vi "Legend Palette.vi"(4 "Active Plot":i32, 6 "Control Ref Queue":T4, 9 "Window Bounds":T5, 10 "Multiplot Representation In":T1, 11 "2D Compass.lvclass in":refnum<class "2D Compass.lvclass">) -> (1 "Cancel?":bool, 2 "Multiplot Representation Out":T1, 3 "2D Compass.lvclass out":refnum<class "2D Compass.lvclass">)   [LabVIEW 2017, in "2D Compass.lvclass"]
uses:
  <vilib>/Math Plots/2D Math Plots/2D Compass/2D Compass/2D Compass.lvclass
  e:/builds/penguin/labview/branches/2017/dev/dist/vi.lib/Math Plots/2D Math Plots/2D Plot/2D Plot/2D Plot.lvclass
  <vilib>/Math Plots/2D Math Plots/2D Plot/Action String/2DMathPlot Ctrl Act Queue.ctl
  <vilib>/Math Plots/2D Math Plots/2D Plot/Action String/2DMathPlot Ctrl Act Cluster.ctl
  <vilib>/Math Plots/2D Math Plots/2D Plot/Action String/2DMathPlot State Class.ctl
  <vilib>/Math Plots/2D Math Plots/2D Plot/2D Plot/Typedef/Multiplot Representation.ctl
  <vilib>/Math Plots/2D Math Plots/2D Plot/2D Plot/Typedef/Plot Representation.ctl
  <vilib>/Math Plots/2D Math Plots/2D Plot/2D Plot/Typedef/Range Cluster.ctl
  <vilib>/Utility/miscctls.llb/LVRectTypeDef.ctl
  <vilib>/Math Plots/2D Math Plots/2D Compass/2D Compass/2D Compass.lvclass/2D Compass.ctl
  <vilib>/Math Plots/2D Math Plots/2D Plot/2D Plot/2D Plot.lvclass
panel:
  in  "Tab Control":enum32{"Plot Property", "Input & Output"}(tab)
  in  "Line Width":u16(ring) caption="Line width"
  in  "Line Style":u16(ring) caption="Line style"
  in  "OK":bool
  in  "Cancel":bool
  in  "Compass size":dbl
  in  "Compass Color":u32(colorbox)
  # "Line style"
  # "Line width"
  # "Compass size"
  # "Compass color"
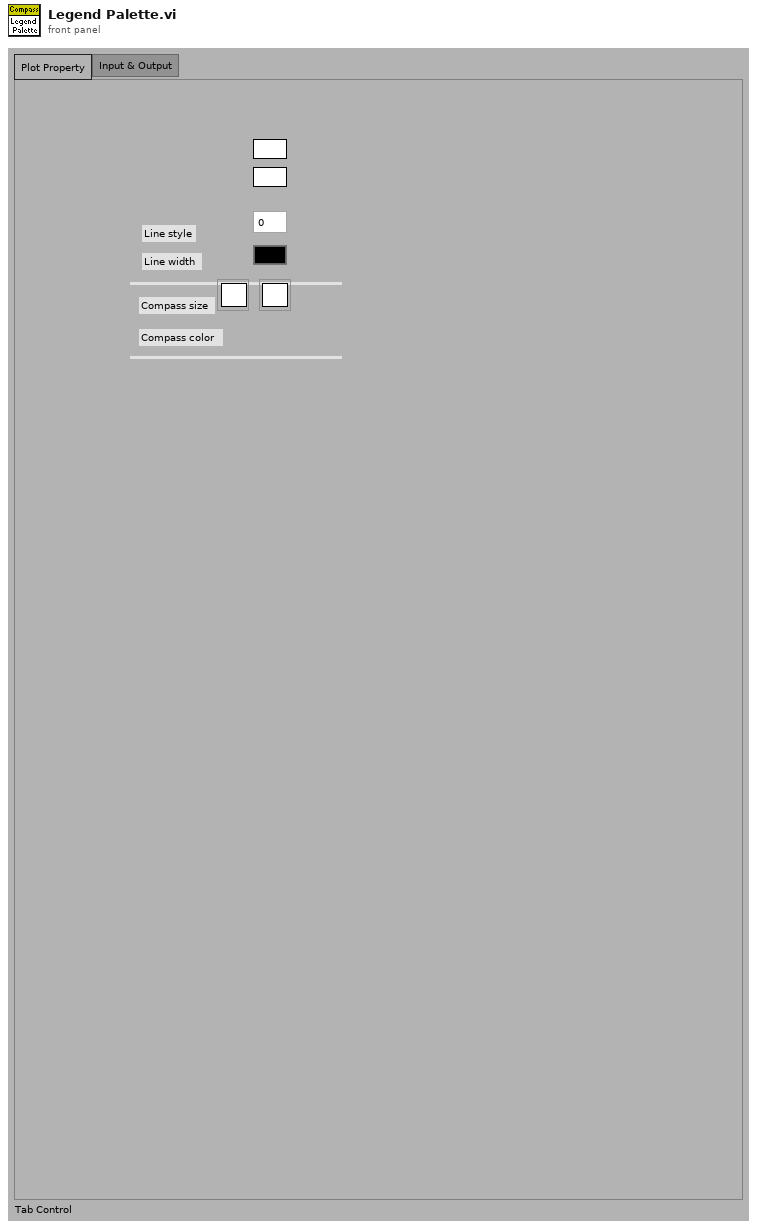
[diagram p1: front panel]
types:
  T1 = typedef "2D Plot.lvclass/Multiplot Representation.ctl" = cluster{"Plot Representation Array":T2[], "Max Range":T3}
  T2 = typedef "2D Plot.lvclass/Plot Representation.ctl" = cluster{"Plot Range":T3, "Vertex Cluster":cluster{"Vertex X Array":dbl[], "Vertex Y Array":dbl[]}, "Base Cluster":cluster{"Base X Array":dbl[], "Base Y Array":dbl[]}}
  T3 = typedef "2D Plot.lvclass/Range Cluster.ctl" = cluster{"X Range":cluster{"Max X":dbl, "Min X":dbl}, "Y Range":cluster{"Max Y":dbl, "Min Y":dbl}}
  T4 = typedef "2DMathPlot Ctrl Act Queue.ctl" = refnum<queue>
  T5 = typedef "LVRectTypeDef.ctl" = cluster{"Left":i16, "Top":i16, "Right":i16, "Bottom":i16}
  T6 = typedef "2DMathPlot Ctrl Act Cluster.ctl" = cluster{"Plot Area Ref":refnum<vi>, "Z Axis Ref":refnum<vi>, "Legend Ref":refnum<vi>, "XControl Ref":refnum<vi>, "Facade Ref":refnum<vi>, "Display State Change Class":T7}
  T7 = typedef "2DMathPlot State Class.ctl" = enum16{"Update All (Undo)", "Update General", "Update Appearance", "Update Format", "Update Scale", "Update Marker", "Update Cursor", "None"}
  T8 = typedef "2D Plot.lvclass/Plot Property Array.ctl" = T9[]
  T9 = typedef "2D Plot.lvclass/Plot Property.ctl" = cluster{"Bar Plot Style":u8, "DigitalLineStyle":u8, "TransitionLocation":u8, "Transition Type":u8, "Fill To":i16, "Fill/Pt. Color":u32, "Label Style":u8, "Line Style":u8, "Line Width":u8, "Plot Color":u32, "Plot Interpolation":u8, "Plot Name":string, "Point Style":u8, "Visible?":bool, "XScaleIdx":u32, "YScaleIdx":u32}
  T10 = typedef "2D Compass.lvclass/2D Compass Property Array.ctl" = T11[]
  T11 = typedef "2D Compass.lvclass/2D Compass Property.ctl" = cluster{"Compass Size":dbl}
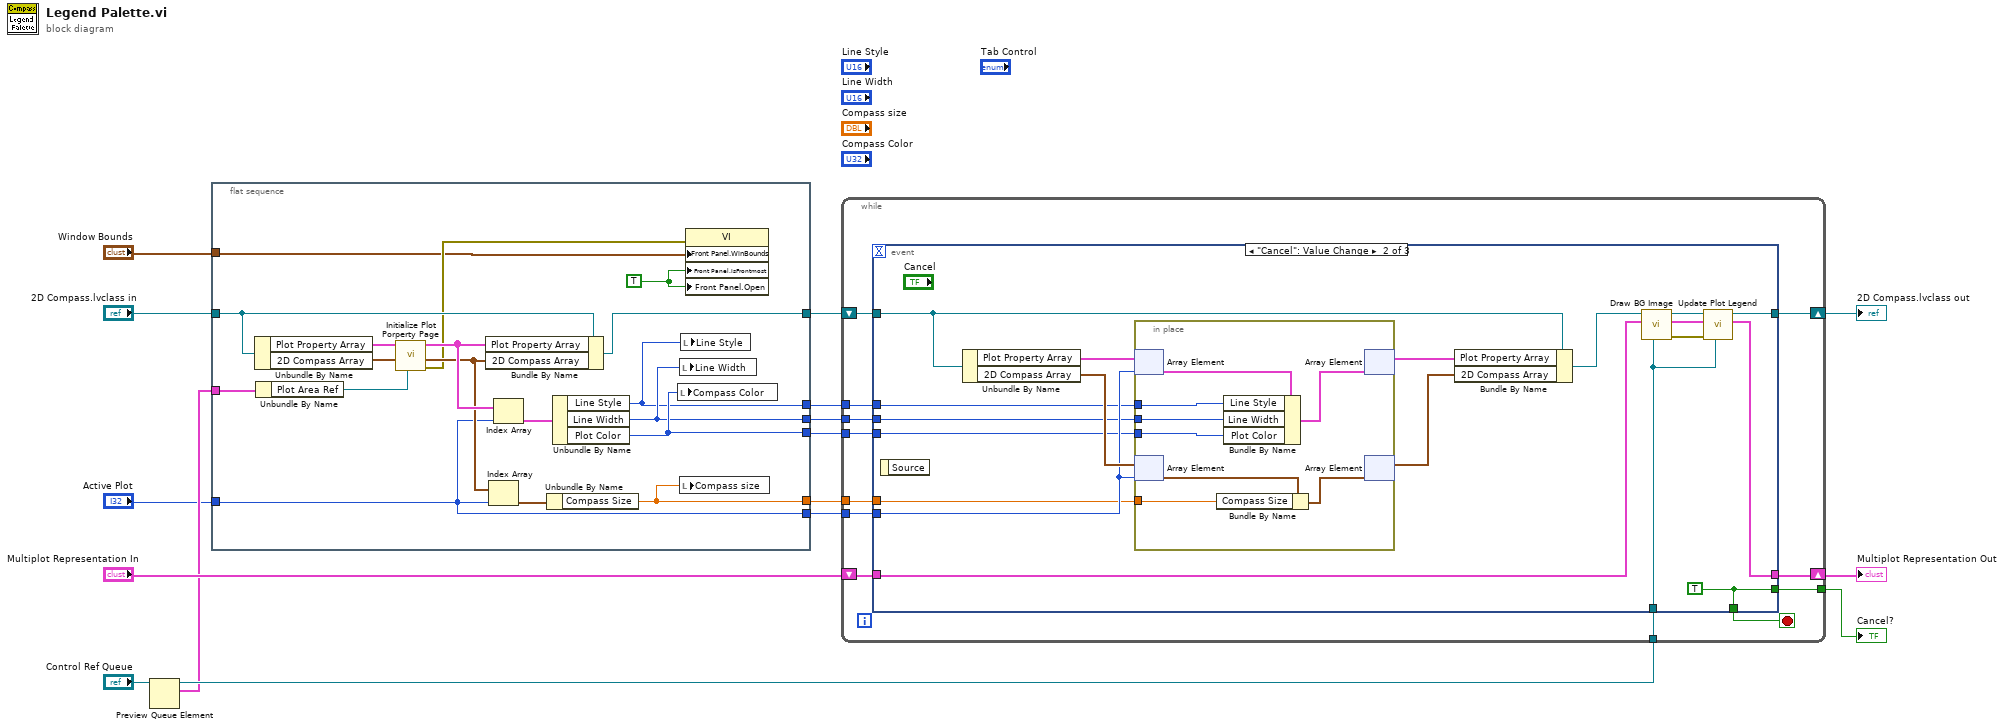
[diagram p0: block diagram]
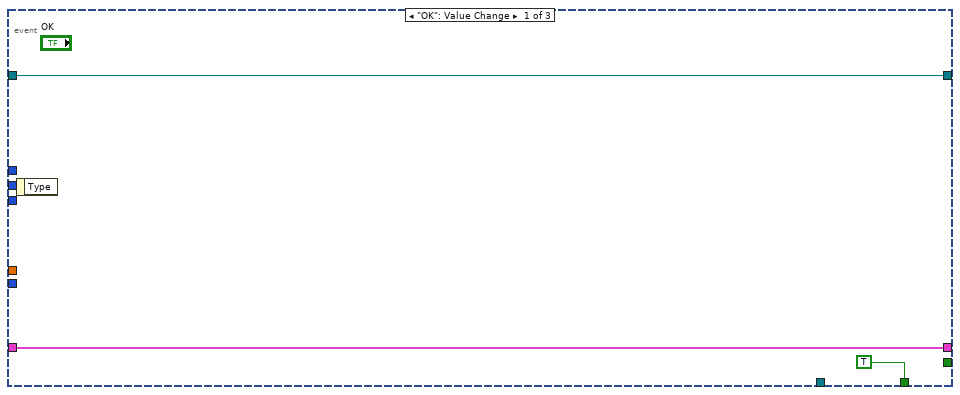
[diagram p2: hidden frame]
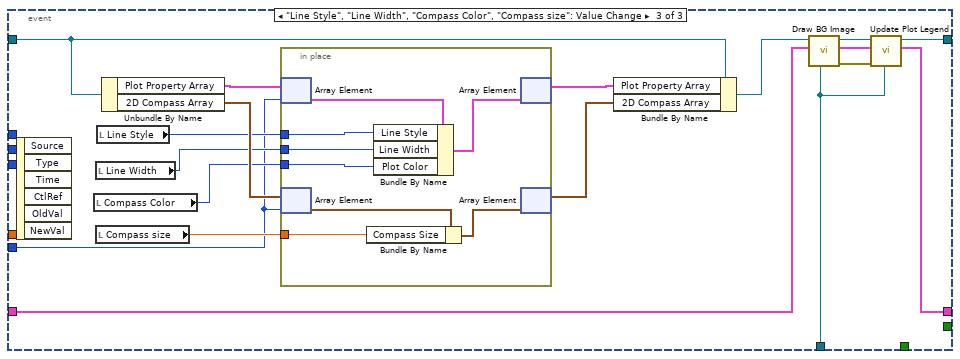
[diagram p3: hidden frame]
diagram:
  n1 = Preview Queue Element(queue="Control Ref Queue") -> (queue out=w10:T4, element=w9:T6)  [unwired: 1 in, 3 out]
  n2 = flat-sequence {
    tunnel: "2D Compass.lvclass in" -> [w21]
    tunnel: [w20] -> w14
    tunnel: [w17] -> w4
    tunnel: w9 -> [w32]
    tunnel: [w30] -> w8
    tunnel: [w29] -> w7
    tunnel: [w28] -> w6
    tunnel: [w27] -> w5
    tunnel: "Window Bounds" -> [w18]
    tunnel: "Active Plot" -> [w17]
    frame #0 {
      w31 = TRUE ("Front Panel Window:Is Frontmost")
      n3 = Unbundle By Name(w21) -> ("Plot Property Array"=w26:T8, "2D Compass Array"=w25:T10)
      n4 = Unbundle By Name(w32) -> ("Plot Area Ref"=w24:refnum<vi>)
      n5 = call <vilib>:"Initialize Plot Porperty Page.vi"("Plot Area Ref"=w24, "2D Compass Array In"=w25, "Plot Property Array In"=w26) -> ("error out"=w19:errorcluster, "2D Compass Array Out"=w22:T10, "Plot Property Array Out"=w23:T8)  [unwired: 2 in, 4 out]
      n6 = Bundle By Name(cluster=w21, "Plot Property Array"=w23, "2D Compass Array"=w22) -> (w20:refnum<class "2D Compass.lvclass">)
      n7 = Index Array(array=w22, index=w17) -> (element=w33:T11)
      n8 = Index Array(array=w23, index=w17) -> (element=w34:T9)
      n9 = Unbundle By Name(w33) -> ("Compass Size"=w30:dbl)
      n10 = Unbundle By Name(w34) -> ("Line Style"=w27:u8, "Line Width"=w28:u8, "Plot Color"=w29:u32)
      n11 = local write "Compass Color"(w29) -> ()
      n12 = local write "Line Width"(w28) -> ()
      n13 = local write "Compass size"(w30) -> ()
      n14 = local write "Line Style"(w27) -> ()
      n15 = property class="VI"(error in=w19, "Front Panel.WinBounds"=w18, "Front Panel.IsFrontmost"=w31, "Front Panel.Open"=w31) -> ()  [unwired: 1 in, 2 out]
    }
  }
  n16 = while {
    shift-right: [w45] -> w16
    shift-left: w14 -> [w46]
    shift-right: [w43] -> w12
    shift-left: "Multiplot Representation In" -> [w44]
    tunnel: w10 -> [w42]
    tunnel: w4 -> [w41]
    tunnel: w8 -> [w39]
    tunnel: w7 -> [w38]
    tunnel: w6 -> [w37]
    tunnel: w5 -> [w36]
    tunnel: [w35] -> w3
    stop <- w40 stop-if-true
    n17 = event shown="[1] \"Cancel\": Value Change" {
      selector: _ -> [_ _ _]
      dyn-events: _ -> [_ _ _]
      timeout: _ -> [_ _ _]
      tunnel: w46 -> [w49 w63 w92]
      tunnel: [w49 w53 w81] -> w45
      tunnel: w44 -> [w48 w62 w84]
      tunnel: [w48 w51 w79] -> w43
      tunnel: w42 -> [_ w52 w78]
      tunnel: w41 -> [_ w61 w83]
      tunnel: [TRUE w50 _] -> w40
      tunnel: w39 -> [_ w60 _]
      tunnel: w38 -> [_ w59 _]
      tunnel: w37 -> [_ w58 _]
      tunnel: w36 -> [_ w57 _]
      tunnel: [_ w50 _] -> w35
      event "OK": Value Change {
        n18 = event-data() -> ()  [unwired: 2 out]
      }
      event "Cancel": Value Change {
        w50 = TRUE
        n19 = event-data() -> ()  [unwired: 2 out]
        n20 = Unbundle By Name(w63) -> ("Plot Property Array"=w68:T8, "2D Compass Array"=w67:T10)
        n21 = in-place {
          in-place-border: w60 -> [w72]
          in-place-border: w57 -> [w71]
          in-place-border: w58 -> [w70]
          in-place-border: w59 -> [w69]
          n22 = in-place-array #1(w68, w61) -> (w76:T9)
          n23 = in-place-array #2(w67, w61) -> (w75:T11)
          n24 = Bundle By Name(cluster=w75, "Compass Size"=w72) -> (w74:T11)
          n25 = Bundle By Name(cluster=w76, "Line Style"=w71, "Line Width"=w70, "Plot Color"=w69) -> (w73:T9)
          n26 = in-place-array #1(w73) -> (w66:T8)  [unwired: 1 out]
          n27 = in-place-array #2(w74) -> (w65:T10)  [unwired: 1 out]
        }
        n28 = Bundle By Name(cluster=w63, "Plot Property Array"=w66, "2D Compass Array"=w65) -> (w64:refnum<class "2D Compass.lvclass">)
        n29 = call-dynamic "Draw BG Image.vi"("Control Ref Queue"=w52, "Multiplot Representation In"=w62, "2D Compass.lvclass in"=w64) -> ("error out"=w54:errorcluster, "Multiplot Representation Out"=w55:T1, "2D Compass.lvclass out"=w56:refnum<class "2D Compass.lvclass">)  [unwired: 1 in, 5 out]
        n30 = call <vilib>:"Update Plot Legend.vi"("Control Ref Queue"=w52, "error in (no error)"=w54, "Multiplot Representation In"=w55, "2D Plot in"=w56) -> ("Multiplot Representation Out"=w51:T1, "2D Plot out"=w53:refnum<class "2D Compass.lvclass">)  [unwired: 6 out]
      }
      event "Line Style", "Line Width", "Compass Color", "Compass size": Value Change {
        n31 = event-data() -> ()  [unwired: 7 out]
        n32 = local read "Compass Color"() -> (w86:u32)
        n33 = local read "Line Width"() -> (w87:u16)
        n34 = local read "Compass size"() -> (w89:dbl)
        n35 = local read "Line Style"() -> (w88:u16)
        n36 = Unbundle By Name(w92) -> ("Plot Property Array"=w94:T8, "2D Compass Array"=w93:T10)
        n37 = in-place {
          in-place-border: w89 -> [w98]
          in-place-border: w88 -> [w97]
          in-place-border: w87 -> [w96]
          in-place-border: w86 -> [w95]
          n38 = in-place-array #3(w94, w83) -> (w102:T9)
          n39 = in-place-array #4(w93, w83) -> (w101:T11)
          n40 = Bundle By Name(cluster=w101, "Compass Size"=w98) -> (w100:T11)
          n41 = Bundle By Name(cluster=w102, "Line Style"=w97, "Line Width"=w96, "Plot Color"=w95) -> (w99:T9)
          n42 = in-place-array #3(w99) -> (w91:T8)  [unwired: 1 out]
          n43 = in-place-array #4(w100) -> (w90:T10)  [unwired: 1 out]
        }
        n44 = Bundle By Name(cluster=w92, "Plot Property Array"=w91, "2D Compass Array"=w90) -> (w85:refnum<class "2D Compass.lvclass">)
        n45 = call-dynamic "Draw BG Image.vi"("Control Ref Queue"=w78, "Multiplot Representation In"=w84, "2D Compass.lvclass in"=w85) -> ("error out"=w77:errorcluster, "Multiplot Representation Out"=w80:T1, "2D Compass.lvclass out"=w82:refnum<class "2D Compass.lvclass">)  [unwired: 1 in, 5 out]
        n46 = call <vilib>:"Update Plot Legend.vi"("Control Ref Queue"=w78, "error in (no error)"=w77, "Multiplot Representation In"=w80, "2D Plot in"=w82) -> ("Multiplot Representation Out"=w79:T1, "2D Plot out"=w81:refnum<class "2D Compass.lvclass">)  [unwired: 6 out]
      }
    }
  }
  "2D Compass.lvclass out" <- w16
  "Multiplot Representation Out" <- w12
  "Cancel?" <- w3
